vi "FindPluginIndex.vi"(8 "error in (no error)":errorcluster, 9 "ItemType":string, 10 "AvailablePluginsNames":string[](array[string]), 11 "SelectedPluginStorage in":refnum<class "SelectedPluginStorage.lvclass">) -> (0 "error out":errorcluster, 2 "PluginIndex":i32, 3 "SelectedPluginStorage out":refnum<class "SelectedPluginStorage.lvclass">)   [LabVIEW 2014, in "SelectedPluginStorage.lvclass"]
uses:
  SelectedPluginStorage.lvclass
  SelectedPluginStorage.lvclass/SelectedPluginStorage.ctl
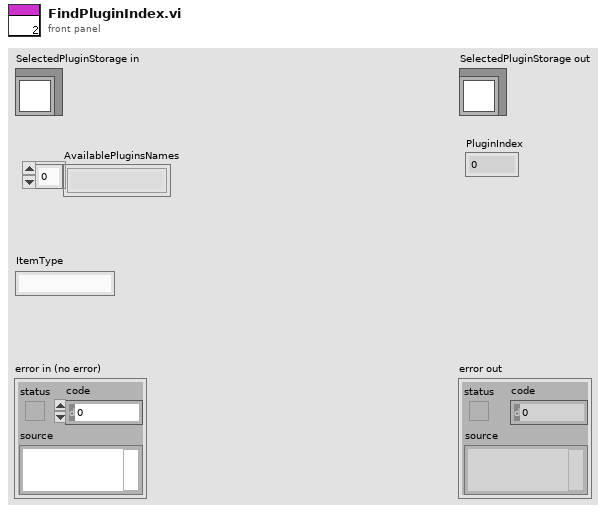
[diagram p1: front panel]
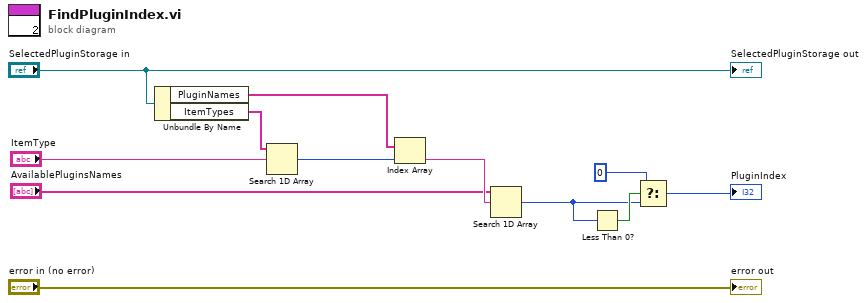
[diagram p0: block diagram]
diagram:
  n1 = Unbundle By Name("SelectedPluginStorage in") -> ("PluginNames"=w8:string[], "ItemTypes"=w9:string[])
  n2 = Search 1D Array(1D array=w9, element="ItemType") -> (index of element=w7:i32)  [unwired: 1 in]
  n3 = Index Array(array=w8, index=w7) -> (element=w6:string)
  n4 = Search 1D Array(1D array="AvailablePluginsNames", element=w6) -> (index of element=w2:i32)  [unwired: 1 in]
  n5 = Less Than 0?(x=w2) -> (x < 0?=w4:bool)
  n6 = Select(t=0, s=w4, f=w2) -> (s? t:f=→"PluginIndex":i32)
  "error out" <- "error in (no error)"
  "SelectedPluginStorage out" <- "SelectedPluginStorage in"
